vi "상태머신.vi"() -> ()   [LabVIEW 2014]
uses:
  Status.ctl
  <vilib>/Analysis/NI_AALBase.lvlib
panel:
  out "웨이브폼 그래프":dbl[](graph)
  in  "확인 버튼":bool
  in  "정지":bool
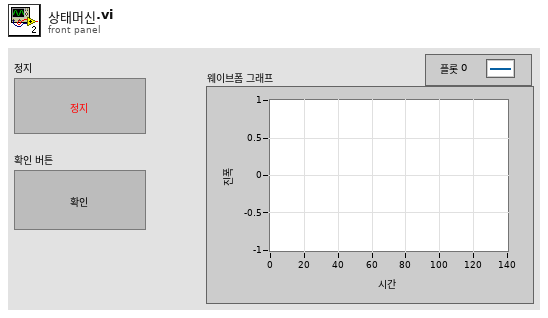
[diagram p1: front panel]
types:
  T1 = typedef "상태머신.ctl" = enum16{"Idle", "초기화", "정지", "Task1", "Task2"}
  T2 = typedef "Status.ctl" = enum16{"Idle", "초기화", "정지", "Task1", "Task2", "Delay", "Task3", "작업4"}
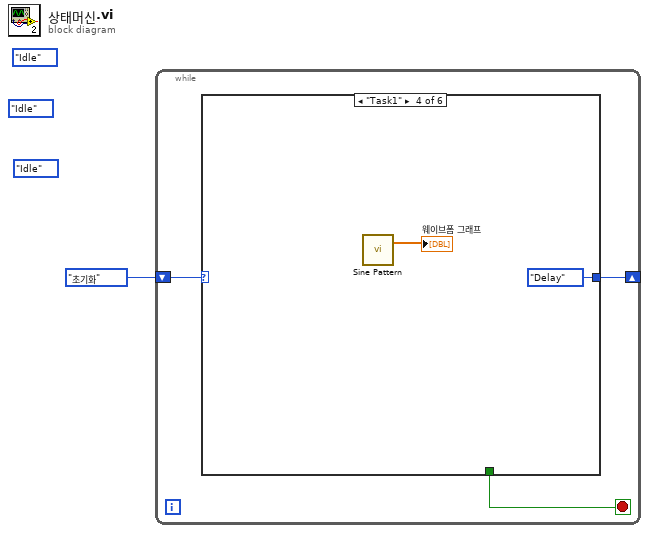
[diagram p0: block diagram]
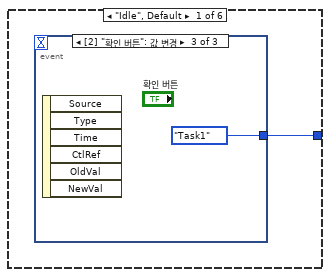
[diagram p2: hidden frame]
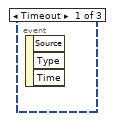
[diagram p3: hidden frame]
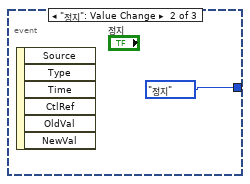
[diagram p4: hidden frame]
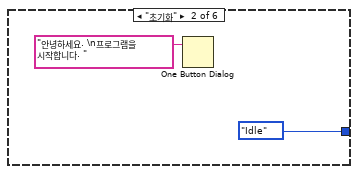
[diagram p5: hidden frame]
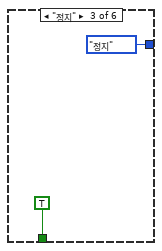
[diagram p6: hidden frame]
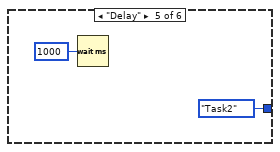
[diagram p7: hidden frame]
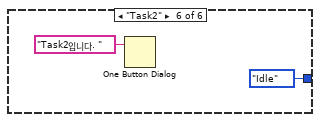
[diagram p8: hidden frame]
diagram:
  (unwired) 상태머신."Idle"
  (unwired) enum16{"Idle", "초기화", "정지"}."Idle"
  (unwired) enum16{"Idle", "초기화", "정지"}."Idle"
  n1 = while {
    shift-right: [w3] -> _
    shift-left: Status."초기화" -> [w4]
    stop <- w2 stop-if-true
    n2 = case shown="\"Task1\"" w4 {
      tunnel: [w5 Status."Idle" Status."정지" Status."Delay" Status."Task2" Status."Idle"] -> w3
      tunnel: [_ _ TRUE _ _ _] -> w2
      frame "Idle", Default {
        n3 = event shown="[2] \"확인 버튼\": 값 변경" {
          selector: _ -> [_ _ _]
          dyn-events: _ -> [_ _ _]
          timeout: _ -> [_ _ _]
          tunnel: [_ Status."정지" Status."Task1"] -> w5
          event Timeout {
            n4 = event-data() -> ()  [unwired: 1 in, 3 out]
          }
          event "정지": Value Change {
            n5 = event-data() -> ()  [unwired: 1 in, 6 out]
          }
          event "확인 버튼": Value Change {
            n6 = event-data() -> ()  [unwired: 1 in, 6 out]
          }
        }
      }
      frame "초기화" {
        n7 = One Button Dialog(message="안녕하세요. \n프로그램을 시작합니다. " ("메시지")) -> ()  [unwired: 1 in, 1 out]
      }
      frame "정지" {
      }
      frame "Task1" {
        n8 = call <vilib>:"Sine Pattern.vi"() -> ("Sinusoidal Pattern"=→"웨이브폼 그래프":dbl[])  [unwired: 4 in, 1 out]
      }
      frame "Delay" {
        n9 = Wait (ms)(milliseconds to wait=u32 1000 ("대기 시간(ms)")) -> ()  [unwired: 1 out]
      }
      frame "Task2" {
        n10 = One Button Dialog(message="Task2입니다. " ("메시지")) -> ()  [unwired: 1 in, 1 out]
      }
    }
  }
